vi "KH_DAQ_FGlob_AI.vi"(5 "Function (Recall One)":T1=enum."Recall one", 7 "PXI_AI_Item 2":i32=2, 8 "err in":errorcluster caption="error", 9 "AI Unscaled IN":i16[](array[numeric]), 10 "AI Values IN":sgl[](array[numeric]) format="%.6f", 11 "StatusIn":bool[](array[boolean])) -> (0 "err out":errorcluster caption="error", 1 "AI Values out unscaled":i16[](array[numeric]), 2 "AI Values OUT":sgl[](array[numeric]) format="%.6f", 3 "StatusOut":bool[](array[boolean]))   [LabVIEW 2021]
uses:
  KH Turck EthernetIP 17.12/KH TURCK TypeDefs FGlob.ctl
panel:
  out "AI Value OUT":sgl format="%.6f"
  in  "AI Value IN":sgl format="%.6f"
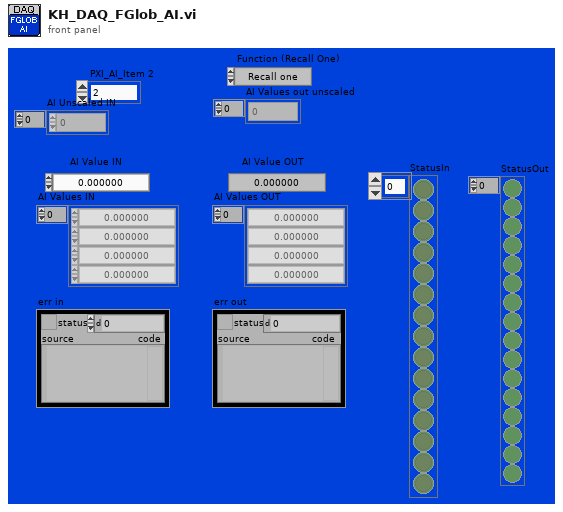
[diagram p1: front panel]
types:
  T1 = typedef "KH TURCK TypeDefs FGlob.ctl" = enum16{"Put one", "Put all", "Recall one", "Recall all"}
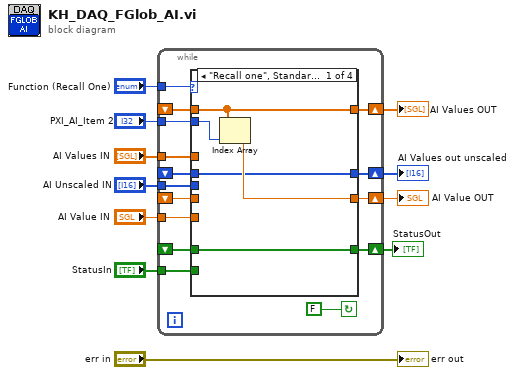
[diagram p0: block diagram]
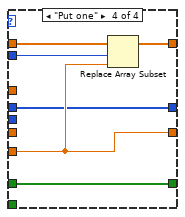
[diagram p4: hidden frame]
diagram:
  n1 = while {
    shift-right: [w25] -> w9
    shift-left: _ -> [w24]
    tunnel: "PXI_AI_Item 2" -> [w22]
    tunnel: "AI Values IN" -> [w21]
    shift-right: [w23] -> w8
    shift-left: _ -> [w20]
    tunnel: "AI Value IN" -> [w19]
    tunnel: "Function (Recall One)" -> [w18]
    shift-right: [w17] -> w4
    shift-left: _ -> [w16]
    tunnel: "AI Unscaled IN" -> [w15]
    tunnel: "StatusIn" -> [w14]
    shift-right: [w13] -> w1
    shift-left: _ -> [w12]
    stop <- FALSE continue-if-true
    n2 = case shown="\"Recall one\", Standard" w18 {
      tunnel: [w29 w35 w38 w44] -> w25
      tunnel: w24 -> [w29 w35 _ w45]
      tunnel: w22 -> [w30 _ _ w43]
      tunnel: [w31 w34 w39 w42] -> w23
      tunnel: w21 -> [_ _ w38 _]
      tunnel: w20 -> [_ w34 w39 _]
      tunnel: w19 -> [_ _ _ w42]
      tunnel: [w28 w33 w37 w41] -> w17
      tunnel: w16 -> [w28 w33 _ w41]
      tunnel: w15 -> [_ _ w37 _]
      tunnel: w14 -> [_ _ w36 _]
      tunnel: [w27 w32 w36 w40] -> w13
      tunnel: w12 -> [w27 w32 _ w40]
      frame "Recall one", Default {
        n3 = Index Array(array=w29, index=w30) -> (element=w31:sgl)
      }
      frame "Recall all" {
      }
      frame "Put all" {
      }
      frame "Put one" {
        n4 = Replace Array Subset(array=w45, new element=w42, index=w43) -> (w44:sgl[])
      }
    }
  }
  "AI Values OUT" <- w9
  "AI Value OUT" <- w8
  "AI Values out unscaled" <- w4
  "StatusOut" <- w1
  "err out" <- "err in"
